vi "Control_3Wheel.vi"(7 "cnt":i32, 10 "input":T1) -> (3 "CMD":cluster{"Tcmd":dbl, "Ocmd":dbl, "itrflg":i32})   [LabVIEW 2013]
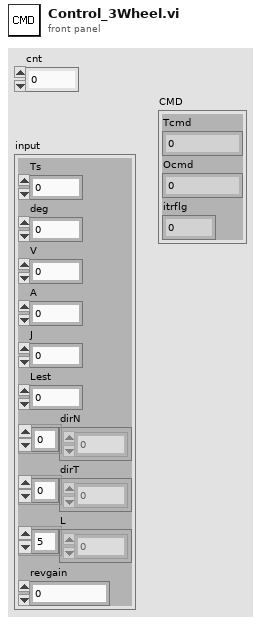
[diagram p1: front panel]
types:
  T1 = cluster{"Ts":dbl, "deg":dbl, "V":dbl, "A":dbl, "J":dbl, "Lest":dbl, "dirN":i32[], "dirT":dbl[], "L":dbl[], "revgain":dbl}
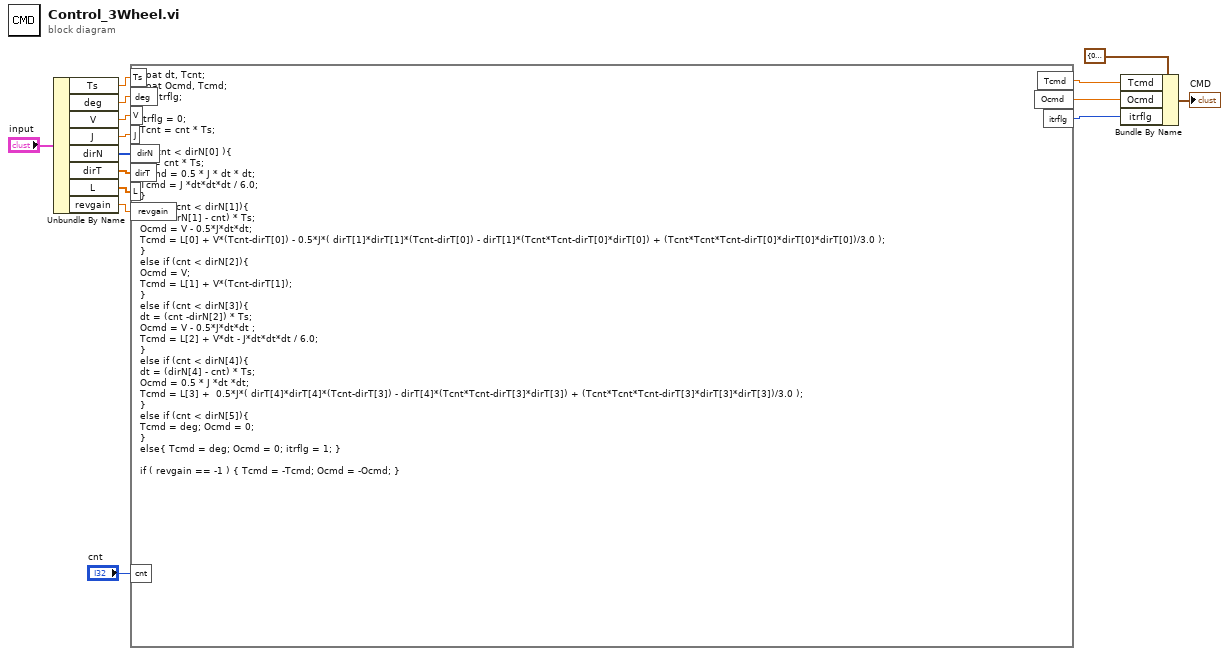
[diagram p0: block diagram]
diagram:
  n1 = Unbundle By Name("input") -> ("Ts"=w11:dbl, "deg"=w12:dbl, "V"=w13:dbl, "J"=w14:dbl, "dirN"=w15:i32[], "dirT"=w9:dbl[], "L"=w8:dbl[], "revgain"=w1:dbl)
  n2 = formula code="float dt, Tcnt;\nfloat Ocmd, Tcmd;\nint itrflg;\n\nitrflg = 0;\nTcnt = cnt * Ts;\n\nif ( cnt < dirN[0] ){\ndt = cnt * Ts; \nOcmd = 0.5 * J * dt * dt;\nTcmd = J *dt*dt*dt / 6.0;\n}\nelse if (cnt < dirN[1]){\ndt = (dirN[1] - cnt) * Ts;\nOcmd = V - 0.5*J*dt*dt;\nTcmd = L[0] + V*(Tcnt-dirT[0]) - 0.5*J*( dirT[1]*dirT[1]*(Tcnt-dirT[0]) - dirT[1]*(Tcnt*Tcnt-dirT[0]*dirT[0]) + (Tcnt*Tcnt*Tcnt-dirT[0]*dirT[0]*dirT[0])/3.0 );\n}\nelse if (cnt < dirN[2]){\nOcmd = V;\nTcmd = L[1] + V*(Tcnt-dirT[1]);\n}\nelse if (cnt < dirN[3]){\ndt = (cnt -dirN[2]) * Ts;\nOcmd = V - 0.5*J*dt*dt ;\nTcmd = L[2] + V*dt - J*dt*dt*dt / 6.0;\n}\nelse if (cnt < dirN[4]){\ndt = (dirN[4] - cnt) * Ts;\nOcmd = 0.5 * J *dt *dt;\nTcmd = L[3] +  0.5*J*( dirT[4]*dirT[4]*(Tcnt-dirT[3]) - dirT[4]*(Tcnt*Tcnt-dirT[3]*dirT[3]) + (Tcnt*Tcnt*Tcnt-dirT[3]*dirT[3]*dirT[3])/3.0 );\n}\nelse if (cnt < dirN[5]){\nTcmd = deg; Ocmd = 0;\n}\nelse{ Tcmd = deg; Ocmd = 0; itrflg = 1; }\n\nif ( revgain == -1 ) { Tcmd = -Tcmd; Ocmd = -Ocmd; }"("cnt"="cnt", "dirN"=w15, "J"=w14, "Ts"=w11, "V"=w13, "deg"=w12, "dirT"=w9, "L"=w8, "revgain"=w1) -> ("Ocmd"=w3:dbl, "Tcmd"=w4:dbl, "itrflg"=w6:i32)
  n3 = Bundle By Name(cluster=cluster{"Tcmd":dbl, "Ocmd":dbl, "itrflg":i32} {"Tcmd"=0.0, "Ocmd"=0.0, "itrflg"=0} ("Cluster"), "Tcmd"=w4, "Ocmd"=w3, "itrflg"=w6) -> (→"CMD":cluster{"Tcmd":dbl, "Ocmd":dbl, "itrflg":i32})
